vi "coTemperatureHumidity.vi"(8 "read buffer":string) -> (9 "h5":dbl, 10 "zone 3":dbl, 11 "h6":dbl caption="h4", 12 "h1":dbl, 13 "h4":dbl, 14 "inlet air":dbl, 15 "h3":dbl, 16 "t1":dbl, 17 "h2":dbl, 18 "t2":dbl, 19 "t5":dbl, 20 "zone 1":dbl, 21 "t6":dbl, 22 "supply":dbl, 23 "t3":dbl, 24 "zone 2":dbl, 25 "t4":dbl, 26 "main return":dbl)   [LabVIEW 2019]
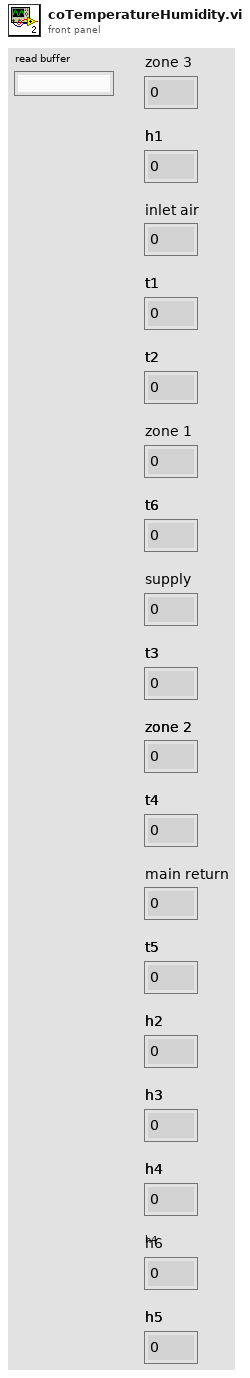
[diagram p1: front panel]
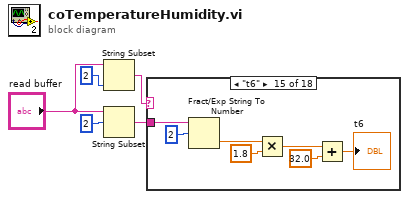
[diagram p0: block diagram]
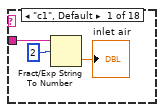
[diagram p2: hidden frame]
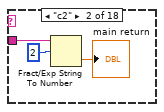
[diagram p3: hidden frame]
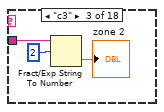
[diagram p4: hidden frame]
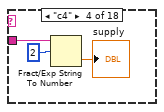
[diagram p5: hidden frame]
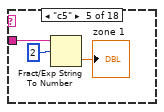
[diagram p6: hidden frame]
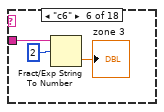
[diagram p7: hidden frame]
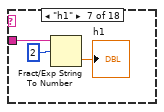
[diagram p8: hidden frame]
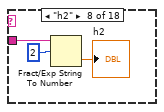
[diagram p9: hidden frame]
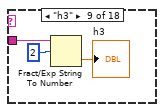
[diagram p10: hidden frame]
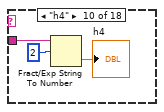
[diagram p11: hidden frame]
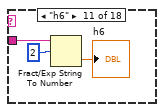
[diagram p12: hidden frame]
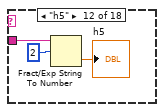
[diagram p13: hidden frame]
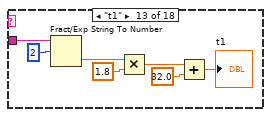
[diagram p14: hidden frame]
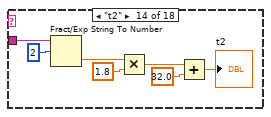
[diagram p15: hidden frame]
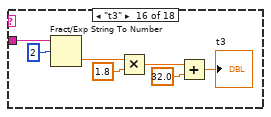
[diagram p16: hidden frame]
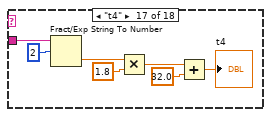
[diagram p17: hidden frame]
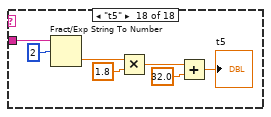
[diagram p18: hidden frame]
diagram:
  n1 = String Subset(string="read buffer", length (rest)=2 ("length (rest)")) -> (substring=w4:string)  [unwired: 1 in]
  n2 = String Subset(string="read buffer", offset (0)=2) -> (substring=w1:string)  [unwired: 1 in]
  n3 = case shown="\"t6\"" w4 {
    tunnel: w1 -> [w7 w10 w13 w16 w19 w22 w25 w28 w31 w34 w37 w40 w47 w54 w61 w68 w75 w82]
    frame "c1", Default {
      n4 = Fract/Exp String To Number(string=w7, offset=2) -> (number=→"inlet air":dbl)  [unwired: 2 in, 1 out]
    }
    frame "c2" {
      n5 = Fract/Exp String To Number(string=w10, offset=2) -> (number=→"main return":dbl)  [unwired: 2 in, 1 out]
    }
    frame "c3" {
      n6 = Fract/Exp String To Number(string=w13, offset=2) -> (number=→"zone 2":dbl)  [unwired: 2 in, 1 out]
    }
    frame "c4" {
      n7 = Fract/Exp String To Number(string=w16, offset=2) -> (number=→"supply":dbl)  [unwired: 2 in, 1 out]
    }
    frame "c5" {
      n8 = Fract/Exp String To Number(string=w19, offset=2) -> (number=→"zone 1":dbl)  [unwired: 2 in, 1 out]
    }
    frame "c6" {
      n9 = Fract/Exp String To Number(string=w22, offset=2) -> (number=→"zone 3":dbl)  [unwired: 2 in, 1 out]
    }
    frame "h1" {
      n10 = Fract/Exp String To Number(string=w25, offset=2) -> (number=→"h1":dbl)  [unwired: 2 in, 1 out]
    }
    frame "h2" {
      n11 = Fract/Exp String To Number(string=w28, offset=2) -> (number=→"h2":dbl)  [unwired: 2 in, 1 out]
    }
    frame "h3" {
      n12 = Fract/Exp String To Number(string=w31, offset=2) -> (number=→"h3":dbl)  [unwired: 2 in, 1 out]
    }
    frame "h4" {
      n13 = Fract/Exp String To Number(string=w34, offset=2) -> (number=→"h4":dbl)  [unwired: 2 in, 1 out]
    }
    frame "h6" {
      n14 = Fract/Exp String To Number(string=w37, offset=2) -> (number=→"h6":dbl)  [unwired: 2 in, 1 out]
    }
    frame "h5" {
      n15 = Fract/Exp String To Number(string=w40, offset=2) -> (number=→"h5":dbl)  [unwired: 2 in, 1 out]
    }
    frame "t1" {
      n16 = Fract/Exp String To Number(string=w47, offset=2) -> (number=w46:dbl)  [unwired: 2 in, 1 out]
      n17 = Multiply(x=w46, y=1.8) -> (x*y=w44:dbl)
      n18 = Add(x=w44, y=32.0) -> (x+y=→"t1":dbl)
    }
    frame "t2" {
      n19 = Fract/Exp String To Number(string=w54, offset=2) -> (number=w53:dbl)  [unwired: 2 in, 1 out]
      n20 = Multiply(x=w53, y=1.8) -> (x*y=w51:dbl)
      n21 = Add(x=w51, y=32.0) -> (x+y=→"t2":dbl)
    }
    frame "t6" {
      n22 = Fract/Exp String To Number(string=w61, offset=2) -> (number=w60:dbl)  [unwired: 2 in, 1 out]
      n23 = Multiply(x=w60, y=1.8) -> (x*y=w58:dbl)
      n24 = Add(x=w58, y=32.0) -> (x+y=→"t6":dbl)
    }
    frame "t3" {
      n25 = Fract/Exp String To Number(string=w68, offset=2) -> (number=w67:dbl)  [unwired: 2 in, 1 out]
      n26 = Multiply(x=w67, y=1.8) -> (x*y=w65:dbl)
      n27 = Add(x=w65, y=32.0) -> (x+y=→"t3":dbl)
    }
    frame "t4" {
      n28 = Fract/Exp String To Number(string=w75, offset=2) -> (number=w74:dbl)  [unwired: 2 in, 1 out]
      n29 = Multiply(x=w74, y=1.8) -> (x*y=w72:dbl)
      n30 = Add(x=w72, y=32.0) -> (x+y=→"t4":dbl)
    }
    frame "t5" {
      n31 = Fract/Exp String To Number(string=w82, offset=2) -> (number=w81:dbl)  [unwired: 2 in, 1 out]
      n32 = Multiply(x=w81, y=1.8) -> (x*y=w79:dbl)
      n33 = Add(x=w79, y=32.0) -> (x+y=→"t5":dbl)
    }
  }
